vi "Initiate Dynamic Waveform.vi"(7 "waveform name (default:\"\")":string="test", 8 "error in (no error)":errorcluster, 9 "Digital Waveform to Generate":digitalwaveform(waveform), 10 "All Pins":string[](array[string])=["CLK", "SDA", "SETID", "VIO", "HV"], 11 "Semiconductor Module Context":T1) -> (0 "error out":errorcluster, 2 "POR Detected":i16, 3 "Acquired Waveform Out":digitalwaveform(waveform)={"t0"=timestamp(0 s since 1904-01-01), "dt"=0.0, "Y"={"transitions"=[], "data"=[]}, "error"={"status"=FALSE, "code"=37421928, "source"=""}}, 6 "Number of Sample Errors Read":i32=6)   [LabVIEW 2013]
doc: "T"
uses:
  <vilib>/NI_TestStand_SemiconductorModule/NI_TestStand_Semiconductor_Module.lvlibp/PinMap/General/SemiconductorModuleContext.ctl
  <vilib>/NI_TestStand_SemiconductorModule/NI_TestStand_Semiconductor_Module.lvlibp/PinMap/General/NIInstrumentTypeIDs.ctl
  <instrlib>/niHSDIO/niHSDIO.llb/niHSDIO_ctl Write Position Values (Ring).ctl
  <vilib>/NI_TestStand_SemiconductorModule/NI_TestStand_Semiconductor_Module.lvlibp/PinMap/HSDIO/PinsToNIHSDIOSessions.vi
  <instrlib>/niHSDIO/niHSDIO.llb/niHSDIO Write Named Waveform (WDT).vi
  <instrlib>/niHSDIO/niHSDIO.llb/niHSDIO Fetch Waveform (WDT).vi
  <vilib>/Waveform/DWDTOps.llb/DWDT Append Digital Signals.vi
  <vilib>/NI_TestStand_SemiconductorModule/NI_TestStand_Semiconductor_Module.lvlibp
panel:
  out "Error Locations":dbl[](array[numeric]) caption="sample numbers"
  out "Digital Waveform Graph":digitalwaveform(graph)={"t0"=timestamp(3403282811.6192408 s since 1904-01-01), "dt"=9.615384615384615e-09, "Y"={"transitions"=[], "data"=[[1, 0, 1, 0], [1, 0, 1, 0], [1, 0, 1, 0], [1, 0, 1, 0], [1, 0, 1, 0], [1, 0, 1, 0], [1, 0, 1, 0], [0, 0, 1, 0], [0, 0, 0, 0], [0, 0, 0, 0], [0, 0, 0, 0], [0, 0, 0, 0], [0, 0, 0, 0], [0, 0, 0, 0], [0, 0, 0, 0], [1, 1, 0, 0], [1, 1, 1, 1], [1, 1, 1, 1], [1, 1, 1, 1], [1, 0, 1, 1], [1, 0, 1, 0], [1, 0, 1, 0], [1, 0, 1, 0], [1, 1, 1, 0], [1, 1, 1, 1], [1, 1, 1, 1], [1, 1, 1, 1], [1, 0, 1, 1], [1, 0, 1, 0], [1, 0, 1, 0], [1, 0, 1, 0], [1, 1, 1, 0], [1, 1, 1, 1], [1, 1, 1, 1], [1, 1, 1, 1], [1, 0, 1, 1], [1, 0, 1, 0], [1, 0, 1, 0], [1, 0, 1, 0], [1, 1, 1, 0], [1, 1, 1, 1], [1, 1, 1, 1], [1, 1, 1, 1], [1, 0, 1, 1], [1, 0, 1, 0], [1, 0, 1, 0], [1, 0, 1, 0], [0, 1, 1, 0], [0, 1, 0, 1], [0, 1, 0, 1], [0, 1, 0, 1], [0, 0, 0, 1], [0, 0, 0, 0], [0, 0, 0, 0], [0, 0, 0, 0], [1, 1, 0, 0], [1, 1, 1, 1], [1, 1, 1, 1], [1, 1, 1, 1], [1, 0, 1, 1], [1, 0, 1, 0], [1, 0, 1, 0], [1, 0, 1, 0], [0, 1, 1, 0], [0, 1, 0, 1], [0, 1, 0, 1], [0, 1, 0, 1], [0, 0, 0, 1], [0, 0, 0, 0], [0, 0, 0, 0], [0, 0, 0, 0], [1, 1, 0, 0], [1, 1, 1, 1], [1, 1, 1, 1], [1, 1, 1, 1], [1, 0, 1, 1], [1, 0, 1, 0], [1, 0, 1, 0], [1, 0, 1, 0], [1, 1, 1, 0], [1, 1, 1, 1], [1, 1, 1, 1], [1, 1, 1, 1], [1, 0, 1, 1], [1, 0, 1, 0], [1, 0, 1, 0], [1, 0, 1, 0], [0, 1, 1, 0], [0, 1, 0, 1], [0, 1, 0, 1], [0, 1, 0, 1], [0, 0, 0, 1], [0, 0, 0, 0], [0, 0, 0, 0], [0, 0, 0, 0], [1, 1, 0, 0], [1, 1, 1, 1], [1, 1, 1, 1], [1, 1, 1, 1], [1, 0, 1, 1], [1, 0, 1, 0], [1, 0, 1, 0], [1, 0, 1, 0], [0, 1, 1, 0], [0, 1, 0, 1], [0, 1, 0, 1], [0, 1, 0, 1], [0, 0, 0, 1], [0, 0, 0, 0], [0, 0, 0, 0], [0, 0, 0, 0], [1, 1, 0, 0], [1, 1, 1, 1], [1, 1, 1, 1], [1, 1, 1, 1], [1, 0, 1, 1], [1, 0, 1, 0], [1, 0, 1, 0], [1, 0, 1, 0], [0, 1, 1, 0], [0, 1, 0, 1], [0, 1, 0, 1], [0, 1, 0, 1], [0, 0, 0, 1], [0, 0, 0, 0], [0, 0, 0, 0], [0, 0, 0, 0], [0, 1, 0, 0], [0, 1, 0, 1], [0, 1, 0, 1], [0, 1, 0, 1], [0, 0, 0, 1], [0, 0, 0, 0], [0, 0, 0, 0], [0, 0, 0, 0], [0, 1, 0, 0], [0, 1, 0, 1], [0, 1, 0, 1], [0, 1, 0, 1], [0, 0, 0, 1], [0, 0, 0, 0], [0, 0, 0, 0], [0, 0, 0, 0], [0, 1, 0, 0], [0, 1, 0, 1], [0, 1, 0, 1], [0, 1, 0, 1], [0, 0, 0, 1], [0, 0, 0, 0], [0, 0, 0, 0], [0, 0, 0, 0], [0, 1, 0, 0], [0, 1, 0, 1], [0, 1, 0, 1], [0, 1, 0, 1], [0, 0, 0, 1], [0, 0, 0, 0], [0, 0, 0, 0], [0, 0, 0, 0], [0, 1, 0, 0], [0, 1, 0, 1], [0, 1, 0, 1], [0, 1, 0, 1], [0, 0, 0, 1], [0, 0, 0, 0], [0, 0, 0, 0], [0, 0, 0, 0], [0, 1, 0, 0], [0, 1, 0, 1], [0, 1, 0, 1], [0, 1, 0, 1], [0, 0, 0, 1], [0, 0, 0, 0], [0, 0, 0, 0], [0, 0, 0, 0], [1, 1, 0, 0], [1, 1, 1, 1], [1, 1, 1, 1], [1, 1, 1, 1], [1, 0, 1, 1], [1, 0, 1, 0], [1, 0, 1, 0], [1, 0, 1, 0], [0, 1, 1, 0], [0, 1, 0, 1], [0, 1, 0, 1], [0, 1, 0, 1], [0, 0, 0, 1], [0, 0, 0, 0], [0, 0, 0, 0], [0, 0, 0, 0], [0, 1, 0, 0], [0, 1, 0, 1], [0, 1, 0, 1], [0, 1, 0, 1], [0, 0, 0, 1], [0, 0, 0, 0], [0, 0, 0, 0], [0, 0, 0, 0], [1, 0, 0, 0], [1, 0, 1, 0], [1, 0, 1, 0], [1, 0, 1, 0], [1, 0, 1, 0], [1, 0, 1, 0], [1, 0, 1, 0], [1, 0, 1, 0], [0, 0, 1, 0], [0, 0, 0, 0], [0, 0, 0, 0], [0, 0, 0, 0], [0, 0, 0, 0], [0, 0, 0, 0], [0, 0, 0, 0], [0, 0, 0, 0], [1, 1, 0, 0], [1, 1, 1, 1], [1, 1, 1, 1], [1, 1, 1, 1], [1, 0, 1, 1], [1, 0, 1, 0], [1, 0, 1, 0], [1, 0, 1, 0], [1, 1, 1, 0], [1, 1, 1, 1], [1, 1, 1, 1], [1, 1, 1, 1], [1, 0, 1, 1], [1, 0, 1, 0], [1, 0, 1, 0], [1, 0, 1, 0], [1, 1, 1, 0], [1, 1, 1, 1], [1, 1, 1, 1], [1, 1, 1, 1], [1, 0, 1, 1], [1, 0, 1, 0], [1, 0, 1, 0], [1, 0, 1, 0], [1, 1, 1, 0], [1, 1, 1, 1], [1, 1, 1, 1], [1, 1, 1, 1], [1, 0, 1, 1], [1, 0, 1, 0], [1, 0, 1, 0], [1, 0, 1, 0], [0, 1, 1, 0], [0, 1, 0, 1], [0, 1, 0, 1], [0, 1, 0, 1], [0, 0, 0, 1], [0, 0, 0, 0], [0, 0, 0, 0], [0, 0, 0, 0], [1, 1, 0, 0], [1, 1, 1, 1], [1, 1, 1, 1], [1, 1, 1, 1], [1, 0, 1, 1], [1, 0, 1, 0], [1, 0, 1, 0], [1, 0, 1, 0], [1, 1, 1, 0], [1, 1, 1, 1], [1, 1, 1, 1], [1, 1, 1, 1], [1, 0, 1, 1], [1, 0, 1, 0], [1, 0, 1, 0], [1, 0, 1, 0], [1, 1, 1, 0], [1, 1, 1, 1], [1, 1, 1, 1], [1, 1, 1, 1], [1, 0, 1, 1], [1, 0, 1, 0], [1, 0, 1, 0], [1, 0, 1, 0], [1, 1, 1, 0], [1, 1, 1, 1], [1, 1, 1, 1], [1, 1, 1, 1], [1, 0, 1, 1], [1, 0, 1, 0], [1, 0, 1, 0], [1, 0, 1, 0], [0, 1, 1, 0], [0, 1, 0, 1], [0, 1, 0, 1], [0, 1, 0, 1], [0, 0, 0, 1], [0, 0, 0, 0], [0, 0, 0, 0], [0, 0, 0, 0], [1, 1, 0, 0], [1, 1, 1, 1], [1, 1, 1, 1], [1, 1, 1, 1], [1, 0, 1, 1], [1, 0, 1, 0], [1, 0, 1, 0], [1, 0, 1, 0], [0, 1, 1, 0], [0, 1, 0, 1], [0, 1, 0, 1], [0, 1, 0, 1], [0, 0, 0, 1], [0, 0, 0, 0], [0, 0, 0, 0], [0, 0, 0, 0], [0, 1, 0, 0], [0, 1, 0, 1], [0, 1, 0, 1], [0, 1, 0, 1], [0, 0, 0, 1], [0, 0, 0, 0], [0, 0, 0, 0], [0, 0, 0, 0], [0, 1, 0, 0], [0, 1, 0, 1], [0, 1, 0, 1], [0, 1, 0, 1], [0, 0, 0, 1], [0, 0, 0, 0], [0, 0, 0, 0], [0, 0, 0, 0], [0, 1, 0, 0], [0, 1, 5, 1], [0, 1, 5, 1], [0, 1, 5, 1], [0, 0, 5, 1], [0, 0, 4, 0], [0, 0, 5, 0], [0, 0, 5, 0], [0, 1, 5, 0], [0, 1, 5, 1], [0, 1, 5, 1], [0, 1, 5, 1], [0, 0, 5, 1], [0, 0, 3, 0], [0, 0, 5, 0], [0, 0, 5, 0], [0, 1, 5, 0], [0, 1, 5, 1], [0, 1, 5, 1], [0, 1, 5, 1], [0, 0, 5, 1], [0, 0, 4, 0], [0, 0, 5, 0], [0, 0, 5, 0], [0, 1, 5, 0], [0, 1, 5, 1], [0, 1, 5, 1], [0, 1, 5, 1], [0, 0, 5, 1], [0, 0, 3, 0], [0, 0, 5, 0], [0, 0, 5, 0], [0, 1, 5, 0], [0, 1, 5, 1], [0, 1, 5, 1], [0, 1, 5, 1], [0, 0, 5, 1], [0, 0, 4, 0], [0, 0, 5, 0], [0, 0, 5, 0], [0, 1, 5, 0], [0, 1, 5, 1], [0, 1, 5, 1], [0, 1, 5, 1], [0, 0, 5, 1], [0, 0, 3, 0], [0, 0, 5, 0], [0, 0, 5, 0], [0, 1, 5, 0], [0, 1, 5, 1], [0, 1, 5, 1], [0, 1, 5, 1], [0, 0, 5, 1], [0, 0, 4, 0], [0, 0, 5, 0], [0, 0, 5, 0], [0, 1, 5, 0], [0, 1, 5, 1], [0, 1, 5, 1], [1, 1, 5, 1], [1, 0, 5, 1], [1, 0, 3, 0], [1, 0, 5, 0], [1, 0, 5, 0], [1, 1, 5, 0], [1, 1, 5, 1], [1, 1, 5, 1], [0, 1, 5, 1], [0, 0, 5, 1], [0, 0, 4, 0], [1, 0, 5, 0], [0, 0, 5, 0], [0, 1, 5, 0], [0, 1, 0, 1], [0, 1, 0, 1], [0, 1, 0, 1], [0, 0, 0, 1], [0, 0, 0, 0], [0, 0, 0, 0], [0, 0, 0, 0], [0, 0, 0, 0]]}}
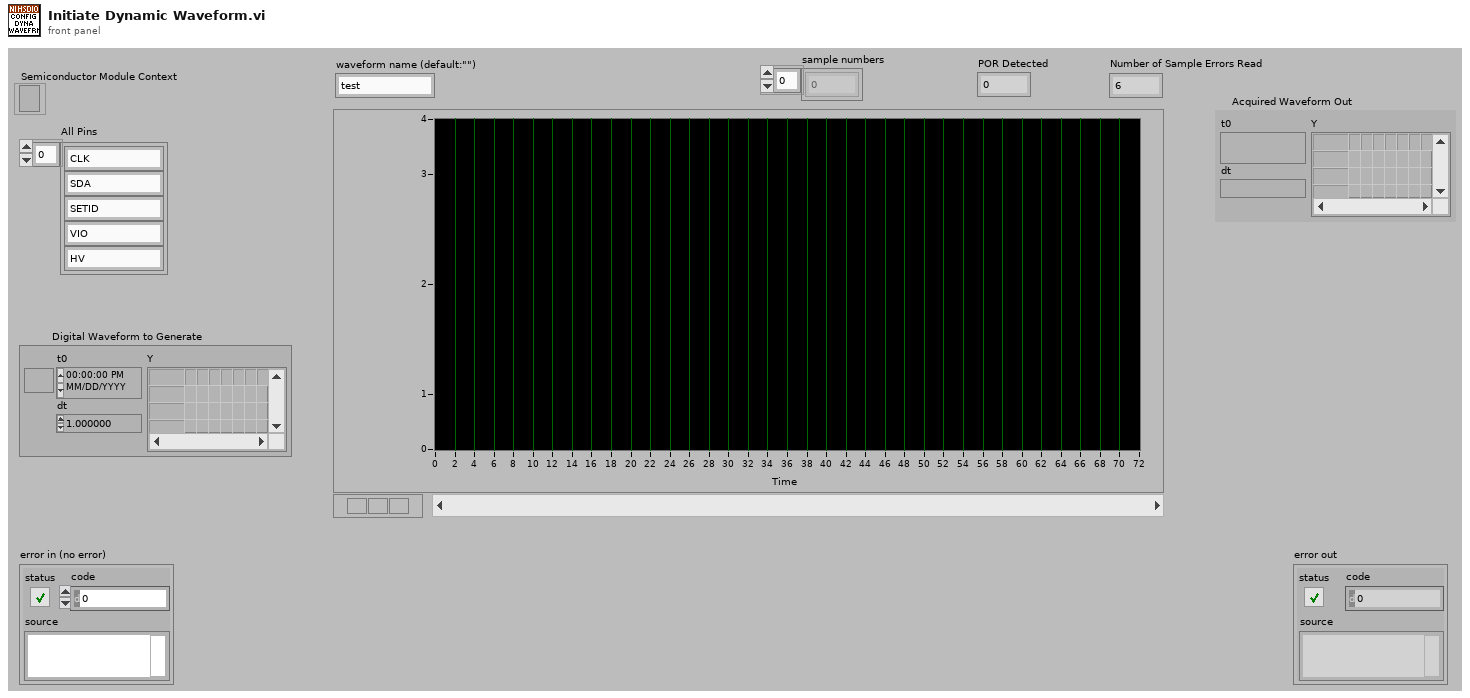
[diagram p1: front panel]
types:
  T1 = typedef "NI_TestStand_Semiconductor_Module.lvlibp/SemiconductorModuleContext.ctl" = refnum<k7>
  T2 = typedef "NI_TestStand_Semiconductor_Module.lvlibp/NIInstrumentTypeIDs.ctl" = string
  T3 = typedef "niHSDIO_ctl Write Position Values (Ring).ctl" = i32
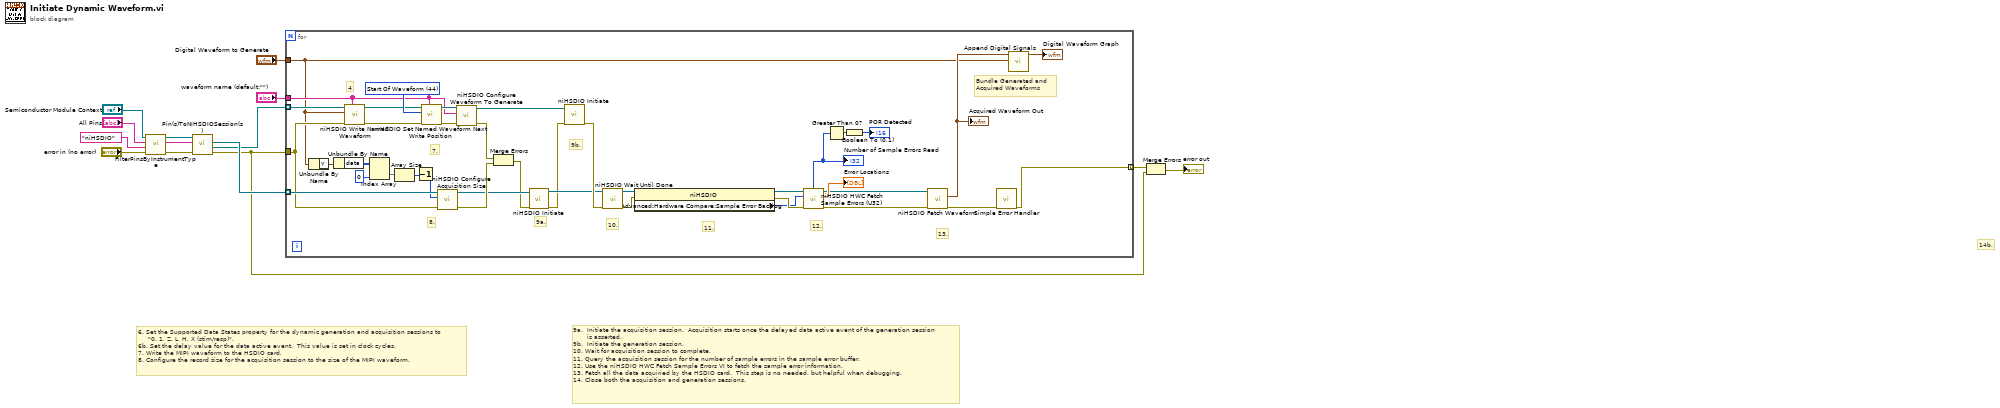
[diagram p0: block diagram]
diagram:
  # "9a.  Initiate the acquisition session.  Acquisition starts once the delayed data active event of the generation session\n       is asserted. \n9b.  Initiate the generation session.\n10. Wait for acquisition session to complete.\n11. Query the acquisition session for the number of sample errors in the sample error buffer.\n12. Use the niHSDIO HWC Fetch Sample Errors VI to fetch the sample error information.\n13. Fetch all the data acquiried by the HSDIO card.  This step is no needed, but helpful when debugging.\n14. Close both the acquisition and generation sessions."
  # "6. Set the Supported Data States property for the dynamic generation and acquisition sessions to \n     \"0, 1, Z, L, H, X (stim/resp)\".\n6b. Set the delay value for the data active event.  This value is set in clock cycles.\n7. Write the MIPI waveform to the HSDIO card.\n8. Configure the record size for the acquisition session to the size of the MIPI waveform."
  # "14b."
  n1 = call <vilib>:"FilterPinsByInstrumentType.vi"("error in (no error)"="error in (no error)", "Instrument Type Id"=T2 "niHSDIO", "Pins"="All Pins", "Semiconductor Module Context"="Semiconductor Module Context") -> ("error out"=w13:errorcluster, "Filtered Pins"=w8:string[], "Semiconductor Module Context Out"=w9:T1)  [unwired: 5 in]
  n2 = call-poly <vilib>:"Pin(s)ToNIHSDIOSession(s).vi"("error in (no error)"=w13, "Pins"=w8, "Semiconductor Module Context"=w9) -> ("error out"=w5:errorcluster, "Generation Sessions"=w6:refnum<k15>[], "Acquisition Sessions"=w7:refnum<k15>[])  [unwired: 3 in, 3 out]
  n3 = for {
    tunnel: w7 -> [w37] mode=indexing
    tunnel: w6 -> [w30] mode=indexing
    tunnel: w5 -> [w31]
    tunnel: [w38] -> w3 mode=indexing
    tunnel: "Digital Waveform to Generate" -> [w18]
    tunnel: "waveform name (default:\"\")" -> [w19]
    w24 = T3 44 items=["Current Write Position"=45, "Start Of Waveform"=44] ("position (current write position)")
    # "4"
    # "Bundle Generated and Acquired Waveforms"
    # "13."
    # "12."
    # "11."
    # "10."
    # "9b."
    # "9a."
    # "8."
    # "7."
    n4 = Unbundle By Name(w18) -> ("Y"=w35:digitaldata)
    n5 = Unbundle By Name(w35) -> ("data"=w32:u8[][])
    n6 = call-poly <instrlib>:"niHSDIO Write Named Waveform.vi"("waveform name (default:\"\")"=w19, "error in (no error)"=w31, "data"=w18, "instrument handle"=w30) -> ("error out"=w23:errorcluster, "instrument handle out"=w20:refnum<k15>)  [unwired: 6 in]
    n7 = Index Array(array=w32, index (col)=0 ("index (row)")) -> (element=w34:u8[])  [unwired: 1 in]
    n8 = Array Size(array=w34) -> (size(s)=w26:i32)
    n9 = Decrement(x=w26) -> (x-1=w25:i32)
    n10 = call <instrlib>:"niHSDIO Set Named Waveform Next Write Position.vi"("waveform name (default:\"\")"=w19, "error in (no error)"=w23, "position (current write position)"=w24, "instrument handle"=w20) -> ("error out"=w22:errorcluster, "instrument handle out"=w21:refnum<k15>)  [unwired: 6 in]
    n11 = call <instrlib>:"niHSDIO Configure Acquisition Size.vi"("error in (no error)"=w31, "samples per record (1000 samples)"=w25, "instrument handle"=w37) -> ("error out"=w49:errorcluster, "instrument handle out"=w48:refnum<k15>)  [unwired: 7 in]
    n12 = call <instrlib>:"niHSDIO Configure Waveform To Generate.vi"("error in (no error)"=w22, "waveform name"=w19, "instrument handle"=w21) -> ("error out"=w29:errorcluster, "instrument handle out"=w28:refnum<k15>)  [unwired: 7 in]
    n13 = Merge Errors(w29, w49) -> (w47:errorcluster)
    n14 = call <instrlib>:"niHSDIO Initiate.vi"("error in (no error)"=w47, "instrument handle"=w48) -> ("error out"=w40:errorcluster, "instrument handle out"=w41:refnum<k15>)  [unwired: 8 in]
    n15 = call <instrlib>:"niHSDIO Initiate.vi"("error in (no error)"=w40, "instrument handle"=w28) -> ("error out"=w43:errorcluster)  [unwired: 8 in, 1 out]
    n16 = call <instrlib>:"niHSDIO Wait Until Done.vi"("error in (no error)"=w43, "instrument handle"=w41) -> ("error out"=w44:errorcluster, "instrument handle out"=w42:refnum<k15>)  [unwired: 8 in]
    n17 = property on="Property Node" class="niHSDIO"(reference=w42, error in=w44) -> (reference out=w45:refnum<k15>, error out=w46:errorcluster, "Advanced:Hardware Compare:Sample Error Backlog"=w39:i32)
    n18 = call <instrlib>:"niHSDIO HWC Fetch Sample Errors (U32).vi"("error in (no error)"=w46, "sample errors  to read"=w39, "instrument handle"=w45) -> ("error out"=w50:errorcluster, "sample numbers"=→"Error Locations":dbl[], "instrument handle out"=w51:refnum<k15>, "number of sample errors read"=w17:i32)  [unwired: 3 in, 2 out]
    "Number of Sample Errors Read" <- w17
    n19 = Greater Than 0?(x=w17) -> (x > 0?=w16:bool)
    n20 = Boolean To (0,1)(Boolean=w16) -> (0, 1=→"POR Detected":i16)
    n21 = call-poly <instrlib>:"niHSDIO Fetch Waveform.vi"("error in (no error)"=w50, "instrument handle"=w51) -> ("error out"=w27:errorcluster, "data"=w36:digitalwaveform)  [unwired: 6 in, 2 out]
    "Acquired Waveform Out" <- w36
    n22 = call <vilib>:"Simple Error Handler.vi"("error in (no error)"=w27) -> ("error out"=w38:errorcluster)  [unwired: 4 in, 4 out]
    n23 = call-poly <vilib>:"Append Digital Signals.vi"("digital waveform (low bits)"=w18, "digital waveform (high bits)"=w36) -> ("digital waveform out"=→"Digital Waveform Graph":digitalwaveform)  [unwired: 8 in, 1 out]
  }
  n24 = Merge Errors(w3, w5) -> (→"error out":errorcluster)
